vi "send_ExptrapolResults_to_AnalysisObj.vi"(0 "SessionID":string, 5 "isotope name":string, 7 "intercept":dbl, 9 "RMSE":dbl, 11 "error in (no error)":errorcluster, 12 "delta-intercept":dbl, 13 "fit type":string) -> (15 "error out":errorcluster)   [LabVIEW 2017]
doc: "sends the ExtrapolationResults (time zero values) to the AnalysisSession (SessionID) and stores them in the ExtrapolResultsArray"
uses:
  Classes/Analysis/Analysis.lvclass
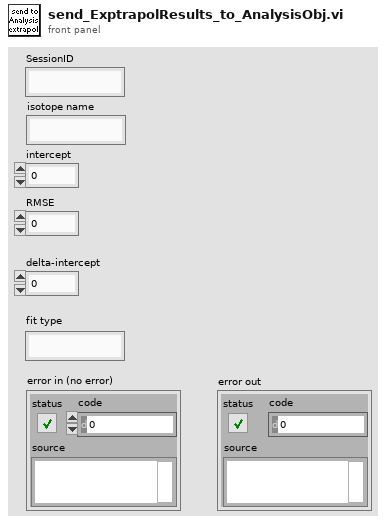
[diagram p1: front panel]
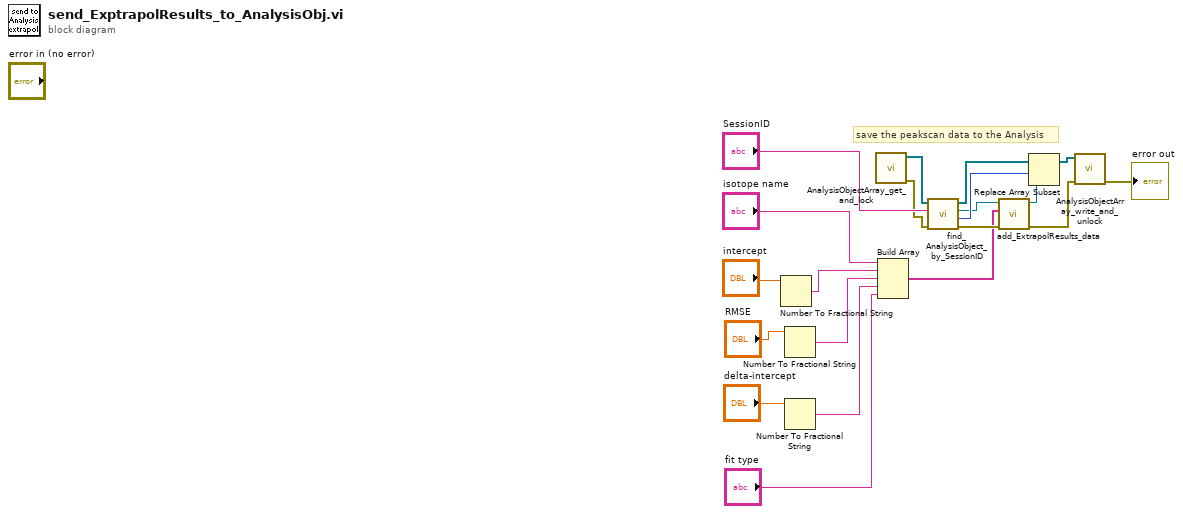
[diagram p0: block diagram]
diagram:
  # "save the peakscan data to the Analysis"
  n1 = Number To Fractional String(number="intercept") -> (F-format string=w6:string)  [unwired: 3 in]
  n2 = Number To Fractional String(number="RMSE") -> (F-format string=w4:string)  [unwired: 3 in]
  n3 = Number To Fractional String(number="delta-intercept") -> (F-format string=w2:string)  [unwired: 3 in]
  n4 = call "AnalysisObjectArray_get_and_lock.vi"() -> ("error out"=w13:errorcluster, "AnalysisObjects"=w10:refnum<class "Analysis.lvclass">[])  [unwired: 10 in]
  n5 = Build Array("isotope name", w6, w4, w2, "fit type") -> (w9:string[])
  n6 = call "find_AnalysisObject_by_SessionID.vi"("error in (no error)"=w13, "SessionID"="SessionID", "AnalysisObjects in"=w10) -> ("error out"=w12:errorcluster, "index of found"=w16:i32, "found AnalyisObject"=w11:refnum<class "Analysis.lvclass">, "AnalysisObjects out"=w14:refnum<class "Analysis.lvclass">[])  [unwired: 5 in]
  n7 = call-dynamic "add_ExtrapolResults_data.vi"("error in (no error)"=w12, "ExtrapolResults"=w9, "Analysis in"=w11) -> ("error out"=w18:errorcluster, "Analysis out"=w15:refnum<class "Analysis.lvclass">)  [unwired: 7 in]
  n8 = Replace Array Subset(array=w14, new element=w15, index=w16) -> (w17:refnum<class "Analysis.lvclass">[])
  n9 = call "AnalysisObjectArray_write_and_unlock.vi"("error in (no error)"=w18, "AnalysisObjects"=w17) -> ("error out"=→"error out":errorcluster)  [unwired: 9 in]
